vi "SetPrior_Zmotor.vi"(0 "object in":refnum<class "Application.lvclass">, 1 "Prior_Zmotor":refnum<class "Prior_Zmotor.lvclass">, 5 "error in (no error)":errorcluster) -> (14 "object out":refnum<class "Application.lvclass">, 19 "error out":errorcluster)   [LabVIEW 2021, in "Application.lvclass"]
uses:
  Application.lvclass
  Application.lvclass/Application.ctl
  Prior_Zmotor_class/Prior_Zmotor.lvclass
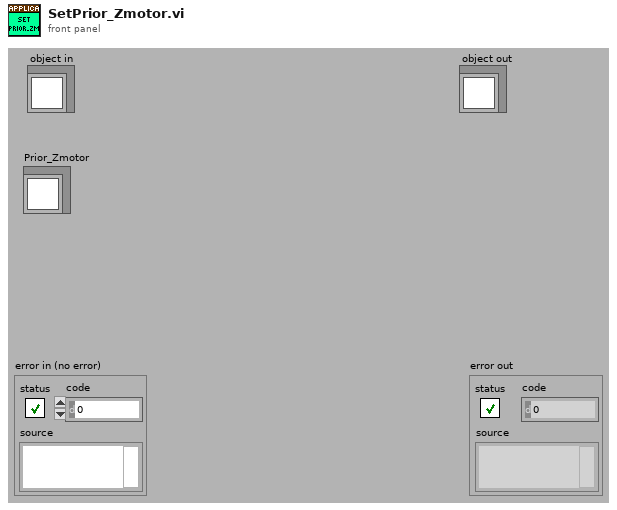
[diagram p1: front panel]
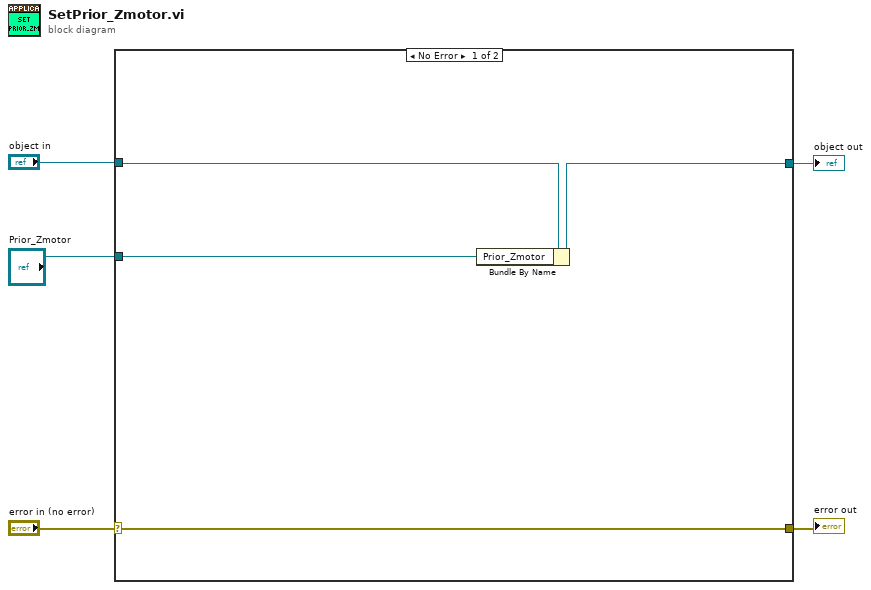
[diagram p0: block diagram]
diagram:
  n1 = case shown="No Error" "error in (no error)" {
    selector: "error in (no error)" -> [w8 w11]
    tunnel: [w8 w11] -> w4
    tunnel: [w6 w10] -> w2
    tunnel: "object in" -> [w7 w10]
    tunnel: "Prior_Zmotor" -> [w9 _]
    frame No Error {
      n2 = Bundle By Name(cluster=w7, "Prior_Zmotor"=w9) -> (w6:refnum<class "Application.lvclass">)
    }
    frame Error {
    }
  }
  "error out" <- w4
  "object out" <- w2
